vi "Read Value.vi"(8 "error in (no error)":errorcluster, 11 "double in":refnum<class "double.lvclass">) -> (0 "error out":errorcluster, 2 "Value":dbl, 3 "double out":refnum<class "double.lvclass">)   [LabVIEW 2020, in "Protobuf RAW.lvlib" / "double.lvclass"]
uses:
  double.lvclass
  double.lvclass/double.ctl
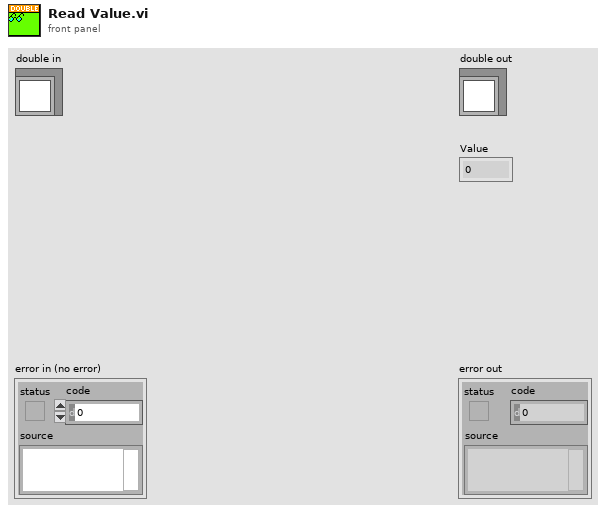
[diagram p1: front panel]
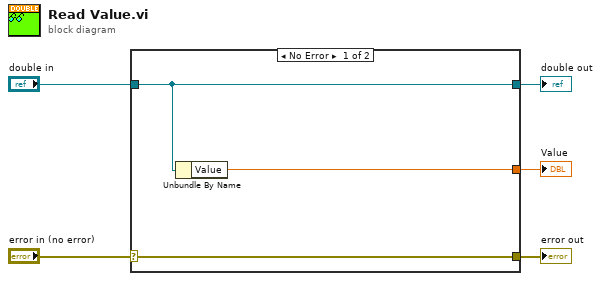
[diagram p0: block diagram]
diagram:
  n1 = case shown="No Error" "error in (no error)" {
    selector: "error in (no error)" -> [w8 w9]
    tunnel: [w8 w9] -> w4
    tunnel: [w7 w10] -> w2
    tunnel: "double in" -> [w7 w10]
    tunnel: [w6 _] -> w1
    frame No Error {
      n2 = Unbundle By Name(w7) -> ("Value"=w6:dbl)
    }
    frame Error {
    }
  }
  "error out" <- w4
  "double out" <- w2
  "Value" <- w1
